vi "xbee_enter_cmode.vi"(8 "error in (no error)":errorcluster, 11 "COM in":refnum<visa-resource-name>) -> (0 "error out":errorcluster, 3 "COM out":refnum<visa-resource-name>)   [LabVIEW 2012]
uses:
  <vilib>/Instr/_visa.llb/VISA Configure Serial Port (Instr).vi
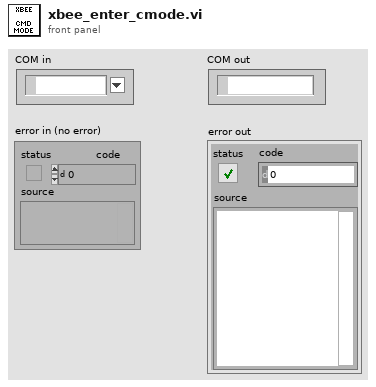
[diagram p1: front panel]
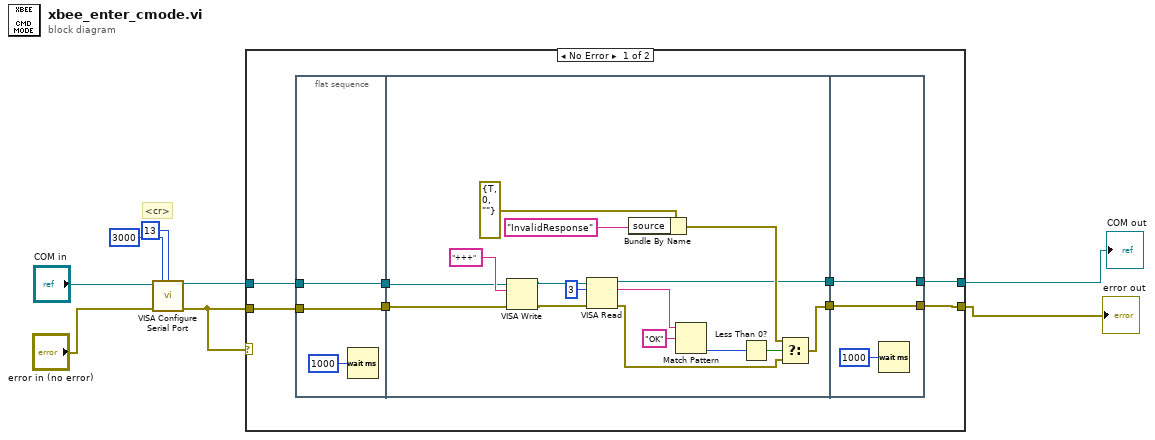
[diagram p0: block diagram]
diagram:
  # "<cr>"
  n1 = call-poly "VISA Configure Serial Port"("VISA resource name"="COM in", "timeout (10sec)"=u32 3000, "termination char\n(0xA = '\\n' = LF)"=u8 13 ("termination char\n(0xA = '\\n' = LF)"), "error in (no error)"="error in (no error)") -> ("VISA resource name out"=w8:refnum<visa-resource-name>, "error out"=w7:errorcluster)  [unwired: 10 in]
  n2 = case shown="No Error" w7 {
    tunnel: w8 -> [w11 w40]
    tunnel: w7 -> [w10 w39]
    tunnel: [w15 w40] -> w1
    tunnel: [w14 w39] -> w6
    frame No Error {
      n3 = flat-sequence {
        tunnel: [w18] -> w12
        tunnel: w11 -> [w18]
        tunnel: w10 -> [w17]
        tunnel: [w17] -> w9
        tunnel: [w23] -> w16
        tunnel: [w22] -> w13
        tunnel: w12 -> [w21]
        tunnel: w9 -> [w20]
        tunnel: [w37] -> w15
        tunnel: w16 -> [w37]
        tunnel: [w36] -> w14
        tunnel: w13 -> [w36]
        frame #0 {
          n4 = Wait (ms)(milliseconds to wait=u32 1000) -> ()  [unwired: 1 out]
        }
        frame #1 {
          n5 = VISA Write(VISA resource name=w21, write buffer="+++", error in (no error)=w20) -> (VISA resource name out=w27:refnum<visa-resource-name>, error out=w28:errorcluster)  [unwired: 1 out]
          n6 = VISA Read(VISA resource name=w27, byte count=u32 3, error in (no error)=w28) -> (VISA resource name out=w23:refnum<visa-resource-name>, read buffer=w30:string, error out=w34:errorcluster)  [unwired: 1 out]
          n7 = Bundle By Name(cluster=errorcluster {"status"=TRUE, "code"=0, "source"=""} ("error constant"), "source"="InvalidResponse") -> (w24:errorcluster)
          n8 = Match Pattern(string=w30, regular expression="OK") -> (offset past match=w32:i32)  [unwired: 1 in, 3 out]
          n9 = Less Than 0?(x=w32) -> (x < 0?=w33:bool)
          n10 = Select(t=w24, s=w33, f=w34) -> (s? t:f=w22:errorcluster)
        }
        frame #2 {
          n11 = Wait (ms)(milliseconds to wait=u32 1000) -> ()  [unwired: 1 out]
        }
      }
    }
    frame Error {
    }
  }
  "error out" <- w6
  "COM out" <- w1
